vi "uObserver_Get_Broker.vi"(8 "error in (no error)":errorcluster, 11 "uObserver in":refnum<class "uObserver.lvclass">) -> (0 "error out":errorcluster, 2 "Broker's Transport":refnum<class "uTransport_uActor.lvclass">, 3 "uObserver out":refnum<class "uObserver.lvclass">)   [LabVIEW 2023, in "uLib.lvlib" / "uObserver.lvclass"]
uses:
  uObserver.lvclass
  uTransport/uTransport_uActor/uTransport_uActor.lvclass
  uObserver.lvclass/uObserver.ctl
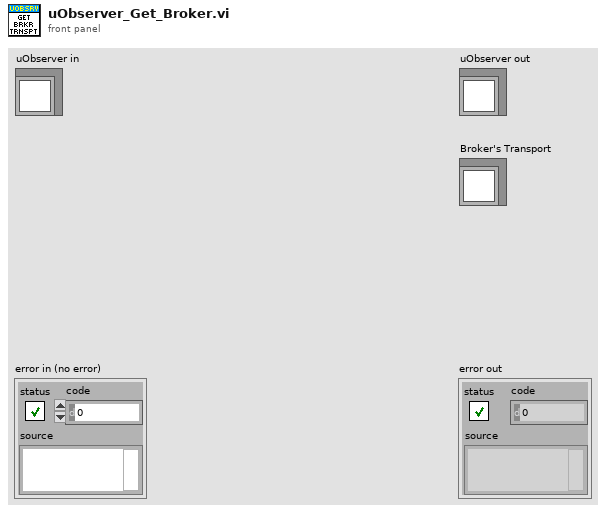
[diagram p1: front panel]
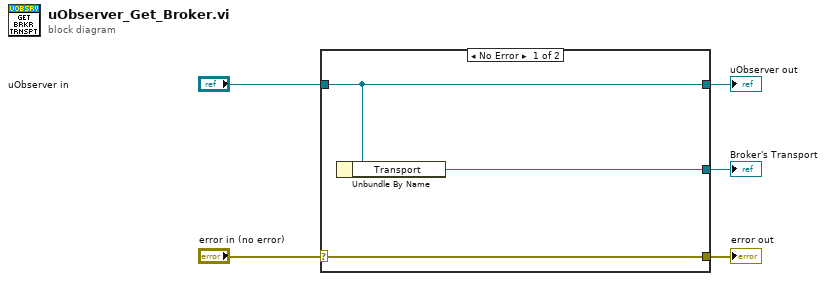
[diagram p0: block diagram]
diagram:
  n1 = case shown="No Error" "error in (no error)" {
    selector: "error in (no error)" -> [w8 w9]
    tunnel: [w8 w9] -> w4
    tunnel: [w7 w10] -> w2
    tunnel: "uObserver in" -> [w7 w10]
    tunnel: [w6 _] -> w1
    frame No Error {
      n2 = Unbundle By Name(w7) -> ("Transport"=w6:refnum<class "uTransport_uActor.lvclass">)
    }
    frame Error {
    }
  }
  "error out" <- w4
  "uObserver out" <- w2
  "Broker's Transport" <- w1
